vi "clase imagini.vi"(11 "dataset folder":path) -> (4 "nume clase":string[](array[string]))   [LabVIEW 2024]
panel:
  # "N-C5p-DataSetTraining"
  # "C:\\proiecte\\lab rn\\L5_BURADA_Rares\\RN-C5_1.bin"
  # "RN-C5_1.bin"
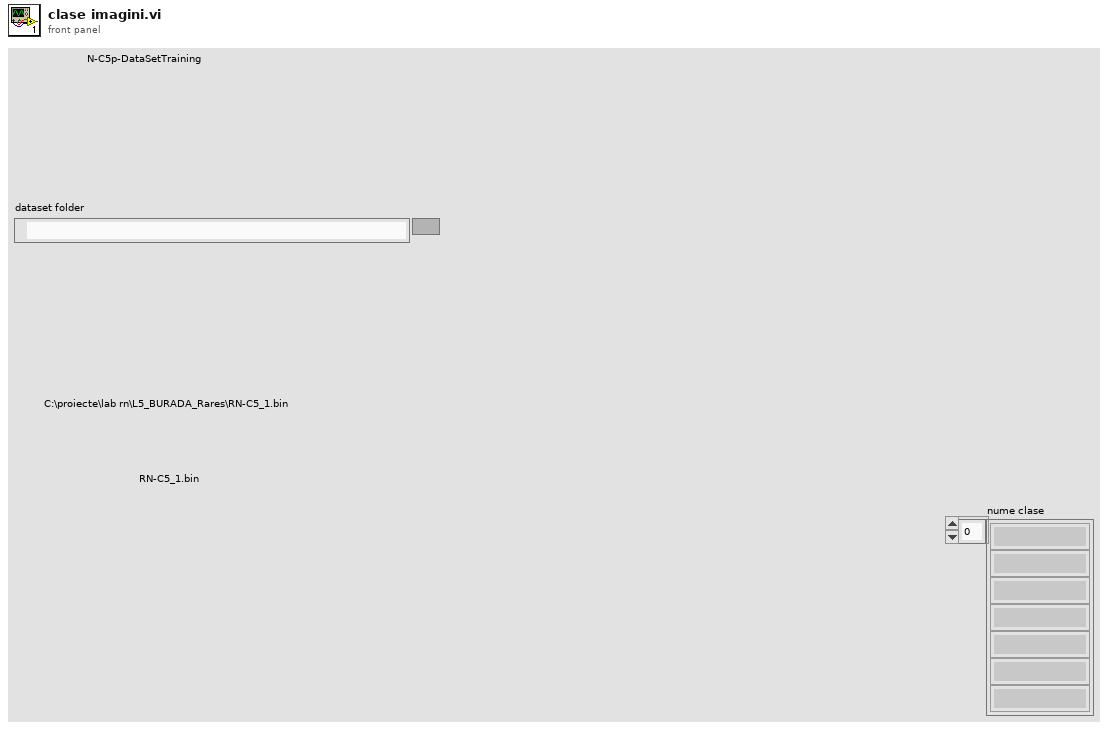
[diagram p1: front panel]
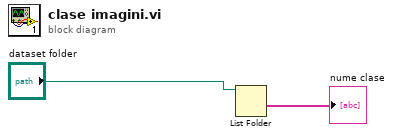
[diagram p0: block diagram]
diagram:
  n1 = List Folder(path="dataset folder") -> (folder names=→"nume clase":string[])  [unwired: 3 in, 3 out]
